vi "3D_template.vi"() -> ()   [LabVIEW 2014]
uses:
  support/Message Queue/Kapitza Message Queue.lvlib
  support/User Event - Stop/Kapitza User Event - Stop.lvlib
  <vilib>/Utility/error.llb/Error Cluster From Error Code.vi
  <vilib>/ErrorRing/Error Ring.xnode
  support/Message Queue/Enqueue Message (Single).vi
  Experiment/Experiment3D/Experiment3D.lvclass
  Measurement/Measurement3D/Measurement3D.lvclass
  Data/Data3D/Data3D.lvclass
  <vilib>/Math Plots/3D Math Plots/3D Surface/3D Surface Datatype/3D Surface Datatype.lvclass
  <vilib>/Math Plots/3D Math Plots/3D Surface/3D Surface Datatype/Public/Plot Helper (Vector).vi
  <vilib>/Math Plots/3D Math Plots/3D Surface/3D Surface XCtrl/3D Surface.xctl
panel:
  in  "Tab Control":enum32{"2D", "3D"}(tab)
  out "XY Graph":cluster{"X":dbl[], "Y":dbl[]}[](graph)
  out "3D Surface":refnum<class "3D Plot Datatype.lvclass">[](xcontrol)
  in  "Max Y":dbl=10.0 caption="Max current Y, uA"
  in  "Step Y":dbl=1.0 caption="Current step Y, uA"
  in  "Init Y":dbl caption="Init current Y, uA"
  in  "Driver 3":path=path "C:/Users/Sergei/YandexDisk/Лаборатория/Projects/Kapitza_prealpha/Drivers/Simulator.vi" caption="Voltmeter driver"
  in  "Address 3":refnum<visa-resource-name> caption="Voltmeter"
  in  "File Path Control":path=path "C:/Users/Sergei/Documents"
  in  "Driver 1":path=path "C:/Users/Sergei/YandexDisk/Лаборатория/Projects/Kapitza_prealpha/Drivers/Simulator.vi" caption="Current source driver"
  in  "Driver 2":path=path "C:/Users/Sergei/YandexDisk/Лаборатория/Projects/Kapitza_prealpha/Drivers/Simulator.vi" caption="Voltmeter driver"
  in  "Address 2":refnum<visa-resource-name> caption="Voltmeter"
  in  "Address 1":refnum<visa-resource-name> caption="Current source"
  in  "Stop":bool
  in  "Sample Name":string="test3D"
  in  "Max X":dbl=10.0 caption="Max current X, uA"
  in  "Step X":dbl=1.0 caption="Current step X, uA"
  in  "Init X":dbl caption="Init current X, uA"
  in  "Start":bool
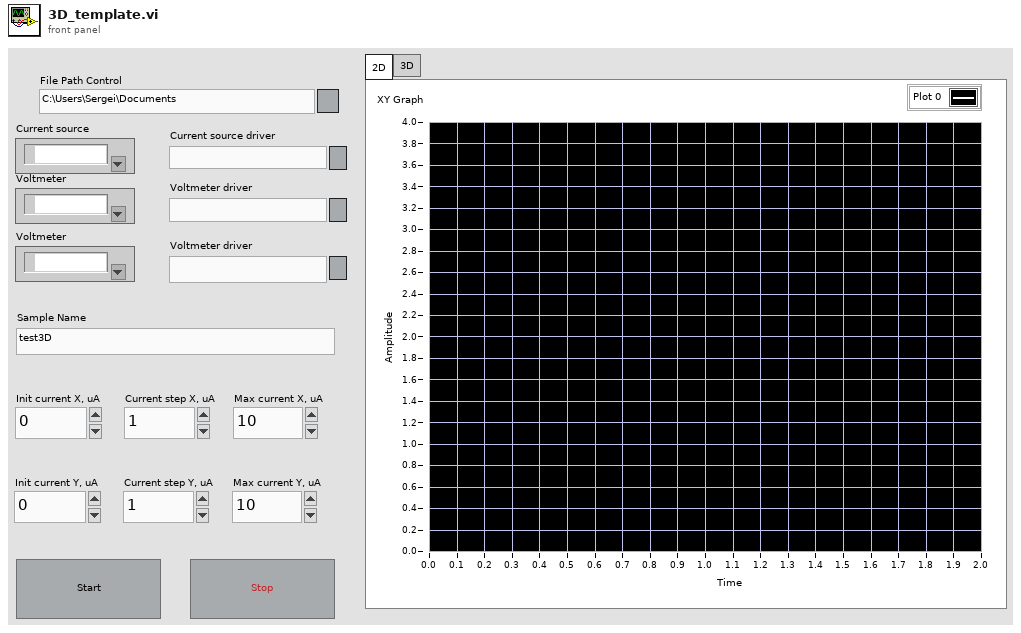
[diagram p1: front panel]
types:
  T1 = typedef "Kapitza Message Queue.lvlib/All Message Queues.ctl" = cluster{"UI":refnum<queue>}
  T2 = cluster{"Init":dbl, "Step":dbl, "Max":dbl, "Current Value":dbl, "Current Index":dbl, "Sweep Outer":dbl[]}
  T3 = cluster{"Init":dbl, "Step":dbl, "Max":dbl, "Current Value":dbl, "Current Index":dbl, "Sweep Inner":dbl[]}
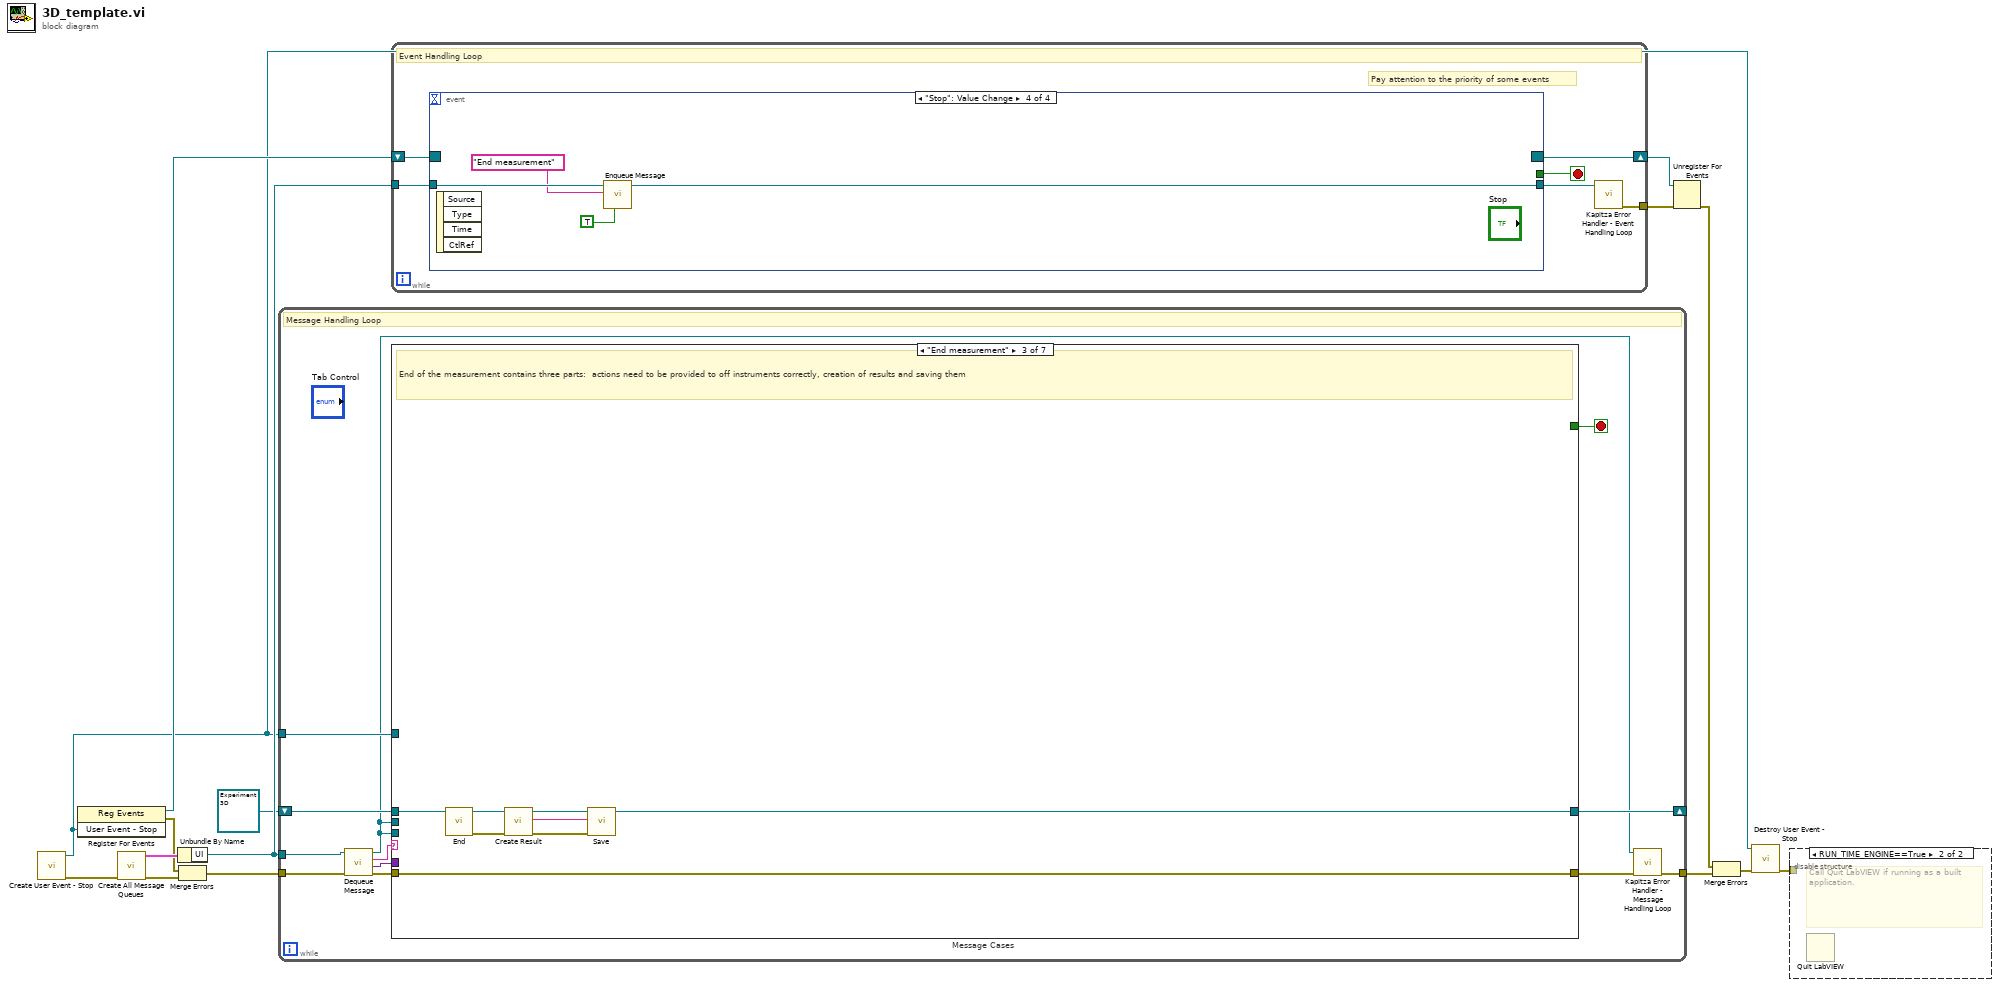
[diagram p0: block diagram]
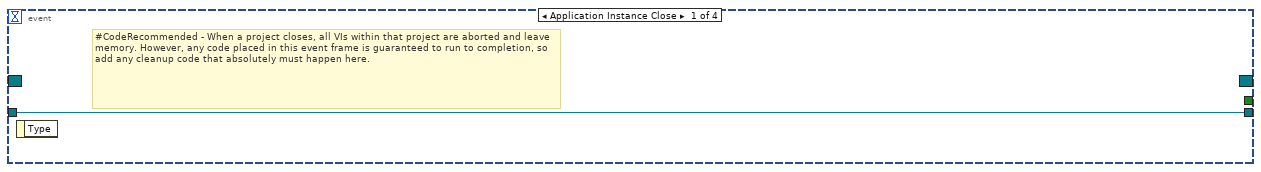
[diagram p3: hidden frame]
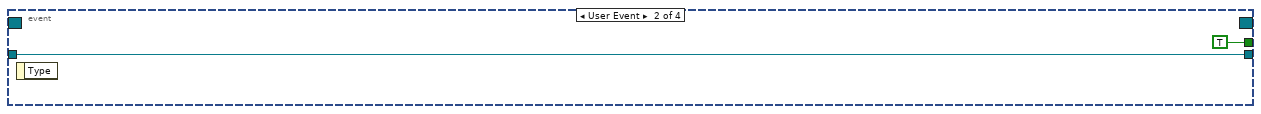
[diagram p4: hidden frame]
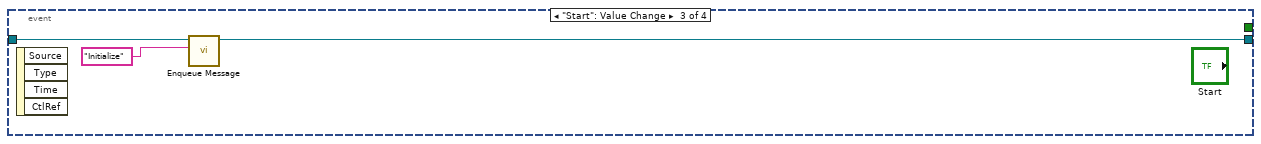
[diagram p5: hidden frame]
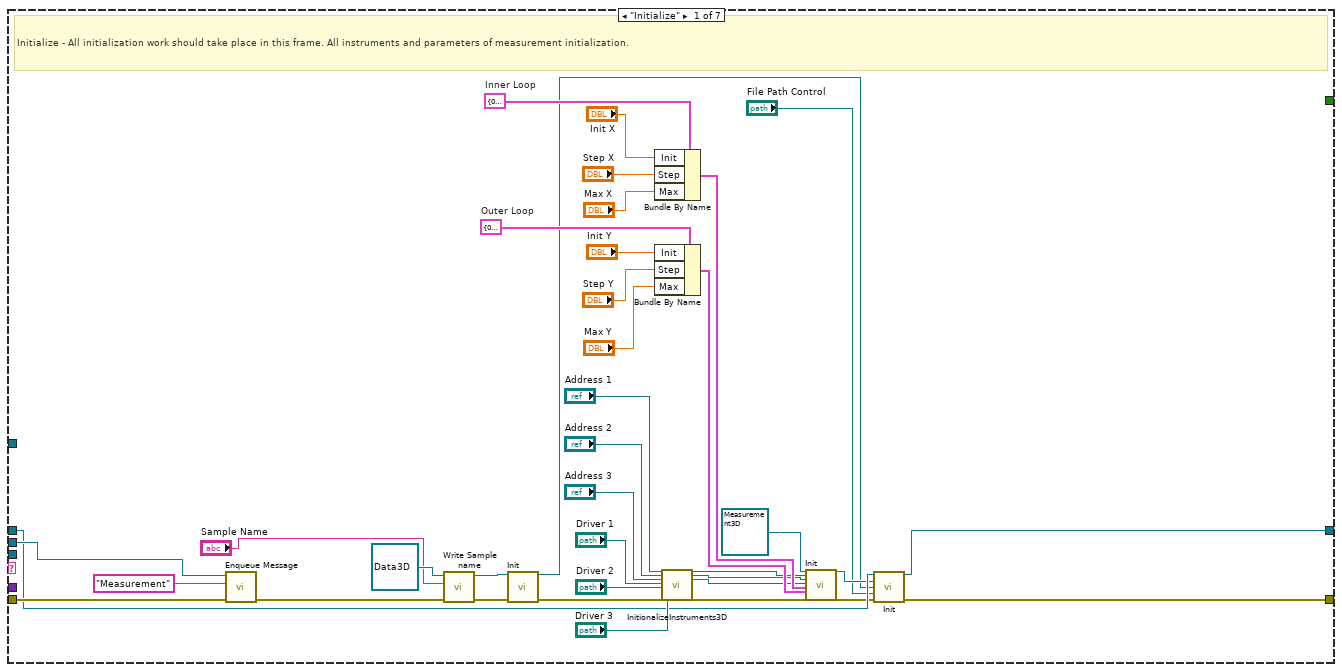
[diagram p6: hidden frame]
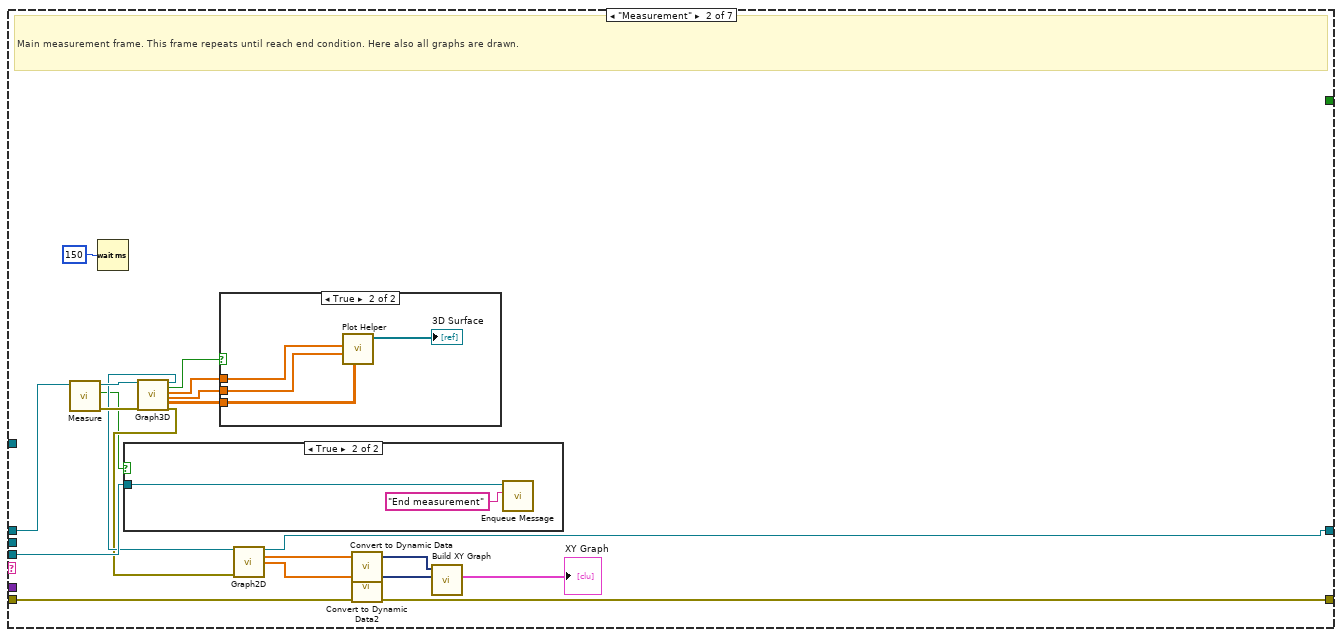
[diagram p7: hidden frame]
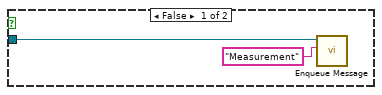
[diagram p8: hidden frame]
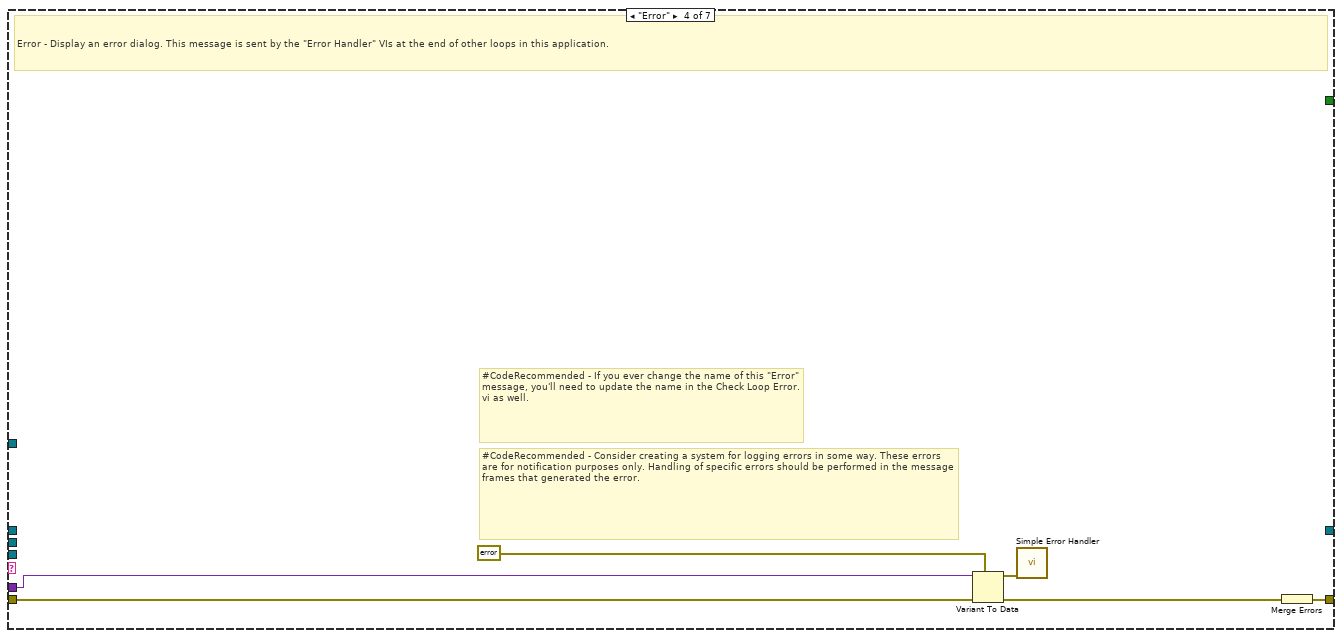
[diagram p10: hidden frame]
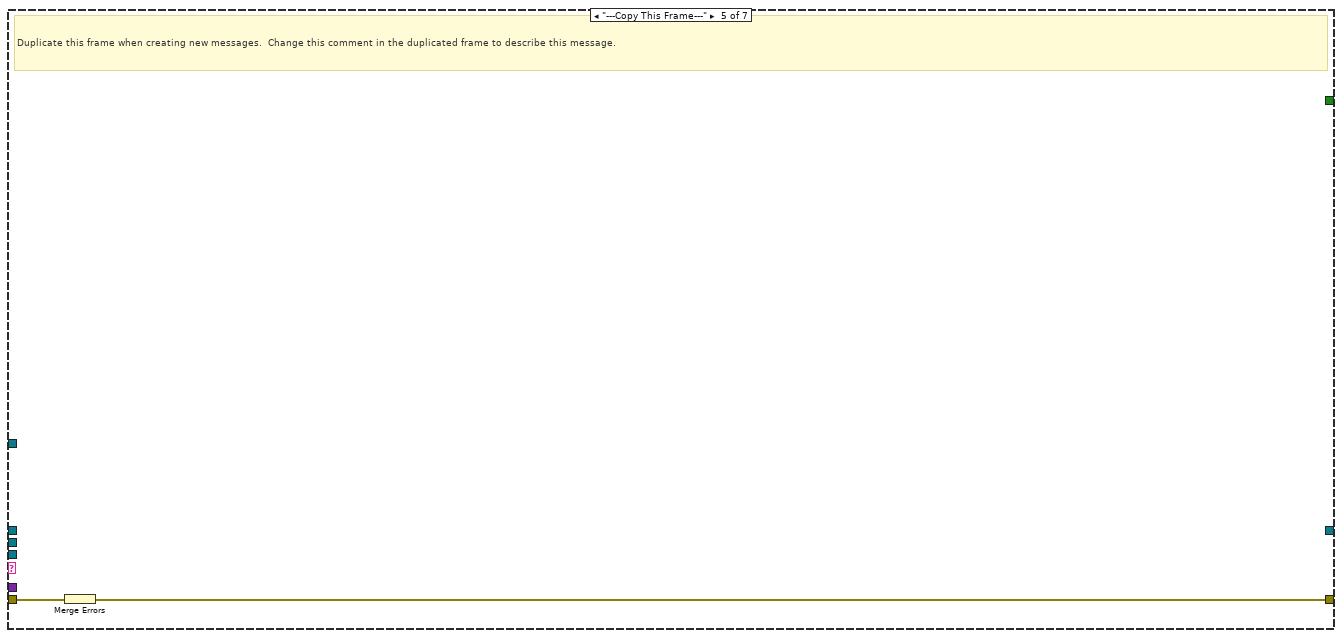
[diagram p11: hidden frame]
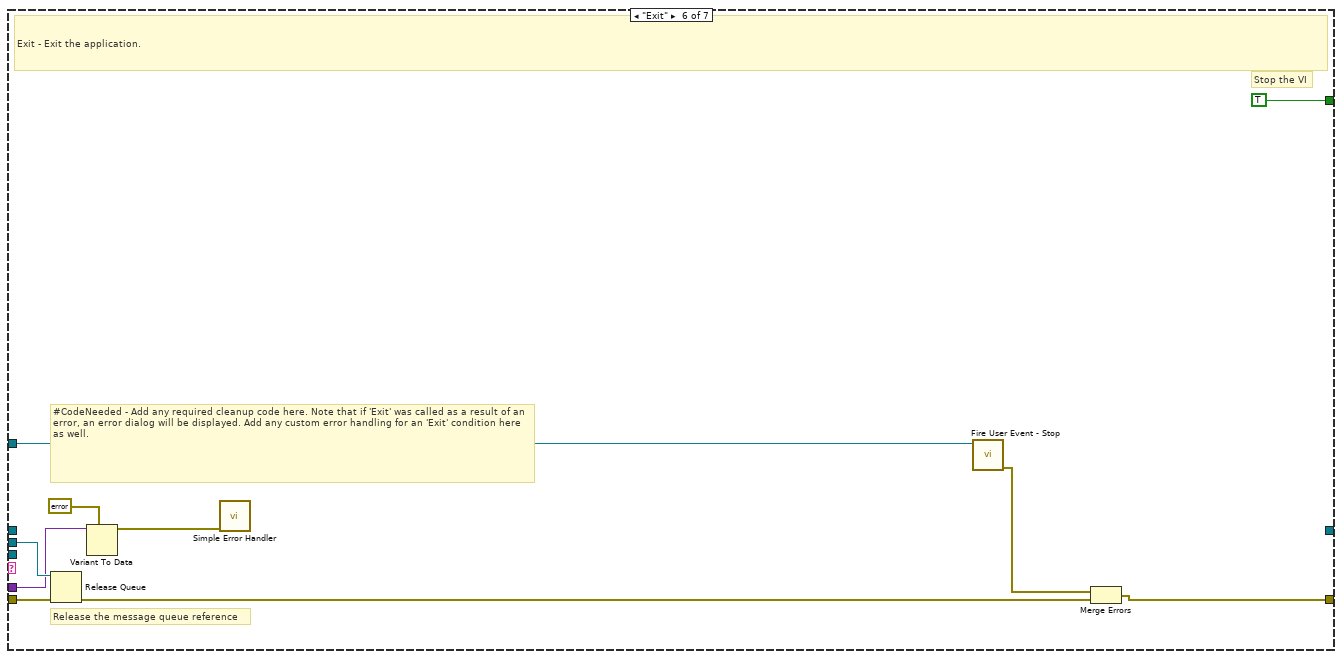
[diagram p12: hidden frame]
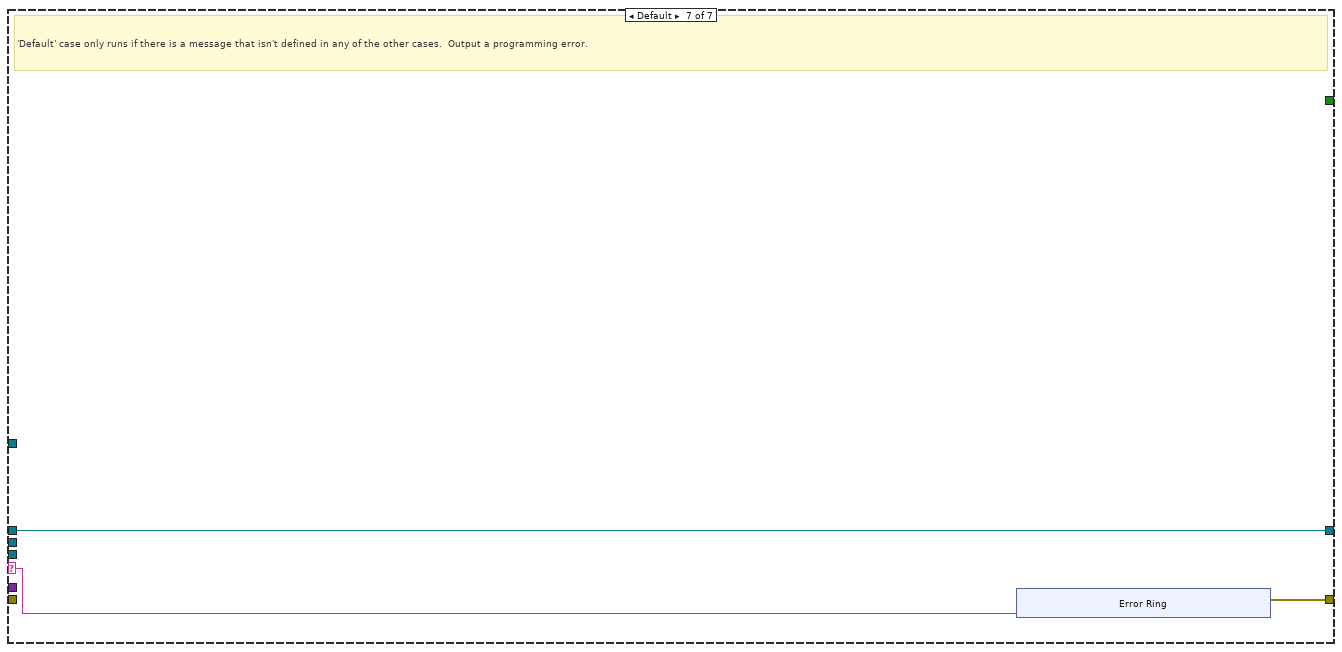
[diagram p13: hidden frame]
diagram:
  n1 = call "Create User Event - Stop.vi"() -> ("error out"=w11:errorcluster, "User Event - Stop"=w4:refnum<user-event>)  [unwired: 10 in]
  n2 = register-events(w4) -> (reference out=w5:refnum<event-registration>, error out=w2:errorcluster)  [unwired: 2 in]
  n3 = call "Create All Message Queues.vi"("error in (no error)"=w11) -> ("error out"=w15:errorcluster, "Message Queues out"=w14:T1)  [unwired: 9 in]
  n4 = Unbundle By Name(w14) -> ("UI"=w12:refnum<queue>)
  n5 = Merge Errors(w2, w15) -> (w3:errorcluster)
  n6 = while {
    tunnel: w12 -> [w21]
    tunnel: w4 -> [w26]
    tunnel: w3 -> [w25]
    tunnel: [w20] -> w13
    shift-right: [w17] -> _
    shift-left: refnum<class "Experiment3D.lvclass"> refnum ("Experiment3D in") -> [w18]
    stop <- w27 stop-if-true
    # "Message Handling Loop"
    n7 = call "Dequeue Message.vi"("error in (no error)"=w25, "Message Queue"=w21) -> ("error out"=w24:errorcluster, "Message Data"=w22:variant, "Message"=w23:string, "dup Message Queue"=w16:refnum<queue>)  [unwired: 6 in]
    n8 = case "Message Cases" shown="\"End measurement\"" w23 {
      selector: w23 -> [_ _ _ _ _ _ w119]
      tunnel: w16 -> [w62 _ _ _ _ w117 _]
      tunnel: w24 -> [w64 w83 w99 w105 w107 w111 _]
      tunnel: [w32 w83 w99 w100 w106 w114 w120] -> w19
      tunnel: [_ _ _ _ _ TRUE _] -> w27
      tunnel: w22 -> [_ _ _ w104 _ w108 _]
      tunnel: w26 -> [_ _ _ _ _ w113 _]
      tunnel: w18 -> [w40 w82 w98 _ _ _ w118]
      tunnel: [w41 w71 w92 _ _ _ w118] -> w17
      tunnel: w16 -> [_ w79 _ _ _ _ _]
      frame "Initialize" {
        w56 = T2 {"Init"=0.0, "Step"=0.0, "Max"=0.0, "Current Value"=0.0, "Current Index"=0.0, "Sweep Outer"=[]}  # Outer Loop
        w61 = T3 {"Init"=0.0, "Step"=0.0, "Max"=0.0, "Current Value"=0.0, "Current Index"=0.0, "Sweep Inner"=[]}  # Inner Loop
        # "Initialize - All initialization work should take place in this frame. All instruments and parameters of measurement initialization."
        n9 = call-poly "Enqueue Message.vi"("error in (no error)"=w64, "Message"="Measurement", "Message Queue"=w62) -> ("error out"=w34:errorcluster)  [unwired: 7 in, 1 out]
        n10 = call "Write Sample name.vi"("error in (no error)"=w34, "Sample name"="Sample Name", "Data3D in"=refnum<class "Data3D.lvclass"> refnum) -> ("error out"=w29:errorcluster, "Data3D out"=w31:refnum<class "Data3D.lvclass">)  [unwired: 7 in]
        n11 = call "Init.vi"("Data3D in"=w31, "error in (no error)"=w29) -> ("Data3D out"=w30:refnum<class "Data3D.lvclass">, "error out"=w28:errorcluster)  [unwired: 12 in]
        n12 = Bundle By Name(cluster=w61, "Init"="Init X", "Step"="Step X", "Max"="Max X") -> (w57:T3)
        n13 = Bundle By Name(cluster=w56, "Init"="Init Y", "Step"="Step Y", "Max"="Max Y") -> (w52:T2)
        n14 = call "InitionalizeInstruments3D.vi"("Address 1"="Address 1", "Address 2"="Address 2", "Address 3"="Address 3", "Driver 1"="Driver 1", "Driver 2"="Driver 2", "error in (no error)"=w28, "Driver 3"="Driver 3") -> ("Instrument out"=w45:refnum<class "Instrument.lvclass">, "Instrument out 2"=w44:refnum<class "Instrument.lvclass">, "Instrument out 3"=w43:refnum<class "Instrument.lvclass">, "error out"=w35:errorcluster)  [unwired: 17 in]
        n15 = call "Init.vi"("Measurement3D in"=refnum<class "Measurement3D.lvclass"> refnum, "Instrument 1.lvclass"=w45, "Instrument 2.lvclass"=w44, "Instrument 3.lvclass"=w43, "Inner Loop"=w57, "Outer Loop"=w52, "error in (no error)"=w35) -> ("Measurement3D out"=w39:refnum<class "Measurement3D.lvclass">, "error out"=w36:errorcluster)  [unwired: 19 in]
        n16 = call "Init.vi"("Experiment3D in"=w40, "Measurement3D.lvclass"=w39, "Data3D.lvclass"=w30, "Path"="File Path Control", "error in (no error)"=w36) -> ("Experiment3D out"=w41:refnum<class "Experiment3D.lvclass">, "error out"=w32:errorcluster)  [unwired: 9 in]
      }
      frame "Measurement" {
        # "Main measurement frame. This frame repeats until reach end condition. Here also all graphs are drawn."
        n17 = call "Measure.vi"("Experiment3D in"=w82) -> ("error out"=w80:errorcluster, "End?"=w65:bool, "Experiment3D out"=w81:refnum<class "Experiment3D.lvclass">)  [unwired: 8 in]
        n18 = Wait (ms)(milliseconds to wait=u32 150) -> ()  [unwired: 1 out]
        n19 = case shown="True" w65 {
          tunnel: w79 -> [w85 w86]
          frame False {
            n20 = call-poly "Enqueue Message.vi"("Message"="Measurement", "Message Queue"=w85) -> ()  [unwired: 8 in, 2 out]
          }
          frame True {
            n21 = call-poly "Enqueue Message.vi"("Message"="End measurement", "Message Queue"=w86) -> ()  [unwired: 8 in, 2 out]
          }
        }
        n22 = call "Graph3D.vi"("Experiment3D in"=w81, "error in (no error)"=w80) -> ("Experiment3D out"=w73:refnum<class "Experiment3D.lvclass">, "Finish?"=w77:bool, "X"=w76:dbl[], "Y"=w75:dbl[], "Z matrix"=w78:dbl[][], "error out"=w72:errorcluster)  [unwired: 12 in]
        n23 = case shown="True" w77 {
          tunnel: w78 -> [_ w91]
          tunnel: w76 -> [_ w89]
          tunnel: w75 -> [_ w88]
          frame False {
          }
          frame True {
            n24 = call-poly <vilib>:"Plot Helper.vi"("z matrix"=w91, "y vector"=w88, "x vector"=w89) -> ("3D Plot lvclass Array out"=→"3D Surface":refnum<class "3D Plot Datatype.lvclass">[])  [unwired: 3 in, 5 out]
          }
        }
        n25 = call "Graph2D.vi"("Experiment3D in"=w73, "error in (no error)"=w72) -> ("Experiment3D out"=w71:refnum<class "Experiment3D.lvclass">, "X-2D"=w69:dbl[], "Y-2D"=w67:dbl[])  [unwired: 10 in, 1 out]
        n26 = call "Convert to Dynamic Data"("Array"=w69) -> ("Dynamic Data Type"=w68:dynamicdata)  [unwired: 3 in]
        n27 = call "Convert to Dynamic Data2"("Array"=w67) -> ("Dynamic Data Type"=w66:dynamicdata)  [unwired: 3 in]
        n28 = call "Build XY Graph"("Y Input"=w66, "X Input"=w68) -> ("XY Graph"=→"XY Graph":cluster{"X":dbl[], "Y":dbl[]}[])  [unwired: 8 in, 1 out]
      }
      frame "End measurement" {
        # "End of the measurement contains three parts:  actions need to be provided to off instruments correctly, creation of results and saving them"
        n29 = call "End.vi"("Experiment3D in"=w98) -> ("error out"=w95:errorcluster, "Experiment3D out"=w97:refnum<class "Experiment3D.lvclass">)  [unwired: 9 in]
        n30 = call "Create Result.vi"("error in (no error)"=w95, "Experiment3D in"=w97) -> ("error out"=w94:errorcluster, "Text"=w96:string, "Experiment3D out"=w93:refnum<class "Experiment3D.lvclass">)  [unwired: 7 in]
        n31 = call "Save.vi"("error in (no error)"=w94, "Text"=w96, "Experiment3D in"=w93) -> ("Experiment3D out"=w92:refnum<class "Experiment3D.lvclass">)  [unwired: 7 in, 1 out]
      }
      frame "Error" {
        # "#CodeRecommended - If you ever change the name of this \"Error\" message, you'll need to update the name in the Check Loop Error.vi as well."
        # "#CodeRecommended - Consider creating a system for logging errors in some way. These errors are for notification purposes only. Handling of specific errors should be performed in the message frames that generated the error."
        # "Error - Display an error dialog. This message is sent by the \"Error Handler\" VIs at the end of other loops in this application."
        n32 = Variant To Data(error in=w105, type=errorcluster {"status"=FALSE, "code"=0, "source"=""} ("error constant"), Variant=w104) -> (data=w102:errorcluster, error out=w101:errorcluster)
        n33 = call <vilib>:"Simple Error Handler.vi"("error in (no error)"=w102) -> ()  [unwired: 4 in, 5 out]
        n34 = Merge Errors(w101) -> (w100:errorcluster)
      }
      frame "---Copy This Frame---" {
        # "Duplicate this frame when creating new messages.  Change this comment in the duplicated frame to describe this message."
        n35 = Merge Errors(w107) -> (w106:errorcluster)
      }
      frame "Exit" {
        # "Stop the VI"
        # "Release the message queue reference"
        # "#CodeNeeded - Add any required cleanup code here. Note that if 'Exit' was called as a result of an error, an error dialog will be displayed. Add any custom error handling for an 'Exit' condition here as well."
        # "Exit - Exit the application."
        n36 = Release Queue(queue=w117, error in (no error)=w111) -> (error out=w115:errorcluster)  [unwired: 1 in, 2 out]
        n37 = Variant To Data(type=errorcluster {"status"=FALSE, "code"=0, "source"=""} ("error constant"), Variant=w108) -> (data=w109:errorcluster)  [unwired: 1 in, 1 out]
        n38 = call <vilib>:"Simple Error Handler.vi"("error in (no error)"=w109) -> ()  [unwired: 4 in, 5 out]
        n39 = call "Fire User Event - Stop.vi"("User Event - Stop"=w113) -> ("error out"=w112:errorcluster)  [unwired: 10 in]
        n40 = Merge Errors(w112, w115) -> (w114:errorcluster)
      }
      frame Default {
        # "'Default' case only runs if there is a message that isn't defined in any of the other cases.  Output a programming error."
        n41 = xnode "Error Ring"("parameter 0"=w119) -> ("error out"=w120:errorcluster)
      }
    }
    n42 = call "Kapitza Error Handler - Message Handling Loop.vi"("error in (no error)"=w19, "Message Queue"=w16) -> ("dup error in"=w20:errorcluster)  [unwired: 8 in, 1 out]
  }
  n43 = while {
    tunnel: w12 -> [w133]
    shift-right: [w131] -> w8
    shift-left: w5 -> [w132]
    tunnel: [w128] -> w6
    stop <- w130 stop-if-true
    # "Pay attention to the priority of some events"
    # "Event Handling Loop"
    n44 = event shown="[3] \"Stop\": Value Change" {
      selector: w132 -> [_ _ _ _]
      dyn-events: [_ _ _ _] -> w131
      timeout: _ -> [_ _ _ _]
      tunnel: [_ TRUE ("Discard?") _ _] -> w130
      tunnel: w133 -> [w134 w136 w139 w143]
      tunnel: [w134 w136 w138 w142] -> w129
      event Application Instance Close {
        # "#CodeRecommended - When a project closes, all VIs within that project are aborted and leave memory. However, any code placed in this event frame is guaranteed to run to completion, so add any cleanup code that absolutely must happen here."
        n45 = event-data() -> ()  [unwired: 1 in, 1 out]
      }
      event User Event {
        n46 = event-data() -> ()  [unwired: 1 in, 1 out]
      }
      event "Start": Value Change {
        n47 = event-data() -> ()  [unwired: 1 in, 4 out]
        n48 = call-poly "Enqueue Message.vi"("Message"="Initialize", "Message Queue"=w139) -> ("dup Message Queue"=w138:refnum<queue>)  [unwired: 8 in, 1 out]
      }
      event "Stop": Value Change {
        n49 = event-data() -> ()  [unwired: 1 in, 4 out]
        n50 = call-poly "Enqueue Message.vi"("Priority Message? (F)"=TRUE, "Message"="End measurement", "Message Queue"=w143) -> ("dup Message Queue"=w142:refnum<queue>)  [unwired: 7 in, 1 out]
      }
    }
    n51 = call "Kapitza Error Handler - Event Handling Loop.vi"("Message Queue"=w129) -> ("dup error in"=w128:errorcluster)  [unwired: 9 in, 1 out]
  }
  n52 = Unregister For Events(event registration refnum=w8, error in=w6) -> (error out=w9:errorcluster)
  n53 = Merge Errors(w9, w13) -> (w10:errorcluster)
  n54 = call "Destroy User Event - Stop.vi"("error in (no error)"=w10, "User Event - Stop"=w4) -> ("error out"=w7:errorcluster)  [unwired: 9 in]
  n55 = disable-structure shown="RUN_TIME_ENGINE==True" {
    disable-tunnel: w7 -> [_ _]
    frame condition #0 (active) {
    }
    frame condition #1 {
      # "Call Quit LabVIEW if running as a built application."
      n56 = Quit LabVIEW() -> ()  [unwired: 1 in]
    }
  }
